vi "Function.vi"(8 "error in (no error)":errorcluster, 9 "Numeric B":dbl, 10 "Numeric A":dbl, 11 "Subtract in":refnum<class "Multiply_DBL.lvclass">) -> (0 "error out":errorcluster, 2 "Result":dbl, 3 "Subtract out":refnum<class "Multiply_DBL.lvclass">)   [LabVIEW 2021, in "Multiply_DBL.lvclass"]
uses:
  Multiply_DBL.lvclass
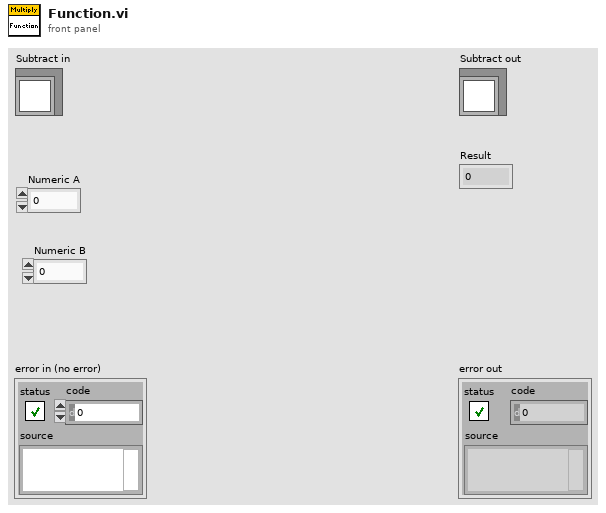
[diagram p1: front panel]
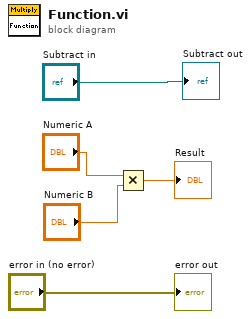
[diagram p0: block diagram]
diagram:
  n1 = Multiply(x="Numeric A", y="Numeric B") -> (x*y=→"Result":dbl)
  "error out" <- "error in (no error)"
  "Subtract out" <- "Subtract in"
